vi "_addrToArray.vi"(11 "addrU32":u32 format="%.0x") -> (3 "addrU8[]LE":u8[](array[numeric]) format="%.0x")   [LabVIEW 2017]
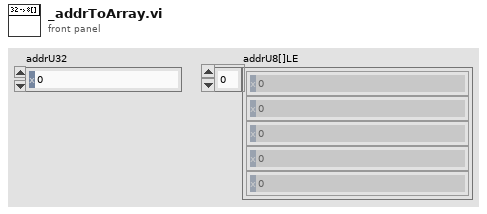
[diagram p1: front panel]
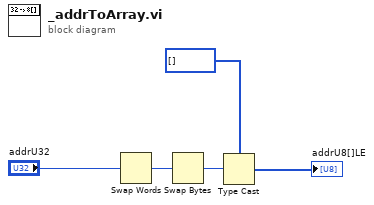
[diagram p0: block diagram]
diagram:
  n1 = Swap Words(1:"addrU32") -> (0:w2:u32)
  n2 = Swap Bytes(anything=w2) -> (byte swapped=w1:u32)
  n3 = Type Cast(type=u8[] [], x=w1) -> (*(type *) &x=→"addrU8[]LE":u8[])
